vi "All Unsafe Config.vi"() -> (2 "All Unsafe Config":T1={"Inspections (All)"=[], "Disallowed ClassNames"=["Open Data Storage", "PathConstant", "Constructor", "Python Node", "Call MATLAB Function"], "Disallowed Functions"=[], "Disallowed SubVI Paths"=[], "Allowed Properties"=["VI Name"], "Allowed Invoke Nodes"=[]})   [LabVIEW 2020, in "SoL Inspector.lvlib"]
uses:
  SoL Inspector.lvlib
  Inspector Config.ctl
  Inspection.ctl
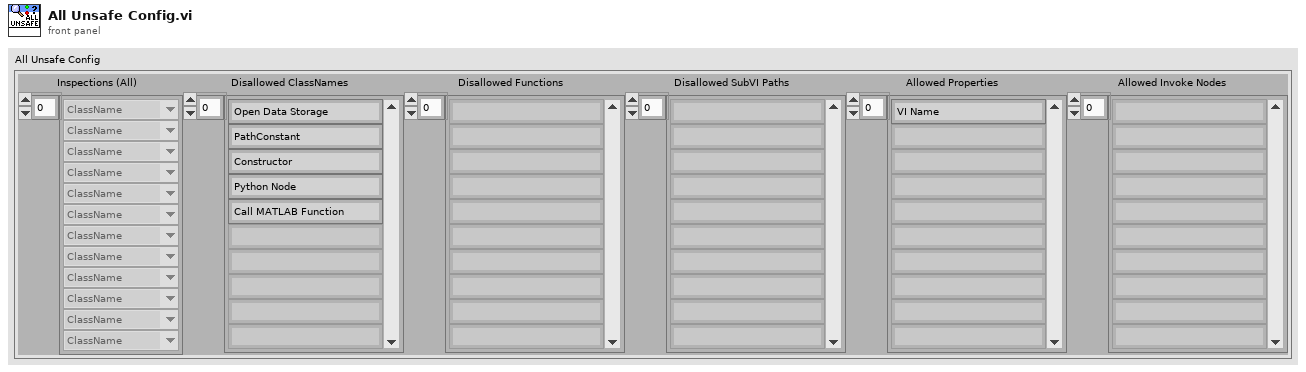
[diagram p1: front panel]
types:
  T1 = typedef "SoL Inspector.lvlib/Inspector Config.ctl" = cluster{"Inspections (All)":T2[], "Disallowed ClassNames":string[], "Disallowed Functions":string[], "Disallowed SubVI Paths":string[], "Allowed Properties":string[], "Allowed Invoke Nodes":string[]}
  T2 = typedef "SoL Inspector.lvlib/Inspection.ctl" = enum16{"ClassName", "Functions", "CallLibrary", "SubVIs", "FileIO", "Invoke Nodes", "Properties", "Growable Functions"}
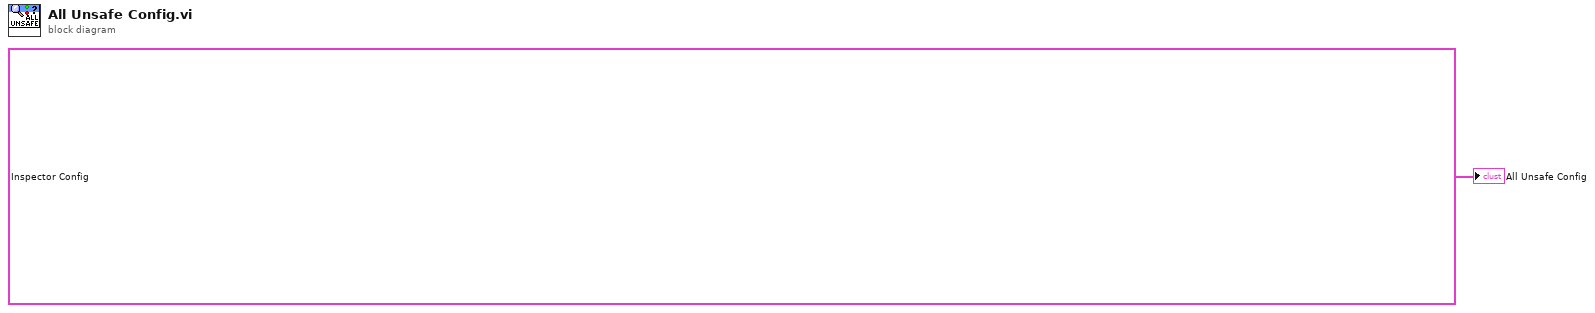
[diagram p0: block diagram]
diagram:
  "All Unsafe Config" <- T1 {"Inspections (All)"=[], "Disallowed ClassNames"=["Open Data Storage", "PathConstant", "Constructor", "Python Node", "Call MATLAB Function"], "Disallowed Functions"=["Open/Create/Replace File", "TCP Open Connection", "Close File", "Read from Binary File", "Write to Binary File", "Read from Text File", "Write to Text File", "TDMS Open", "New VI Object", "Open VI Object Reference", "New VI", "Call Chain", "Quit LabVIEW", "Stop", "Open Application Reference", "Open/Create/Replace Datalog", "Set Type and Creator", "Set File Size", "Set Permissions", "Delete", "Copy", "Move", "File/Directory Info", "Get Volume Info", "List Folder", "Create Folder", "Current VI's Path", "Temporary Directory", "Default Directory", "DataSocket Close", "DataSocket Open", "DataSocket Write", "DataSocket Read", "Create Network Stream Reader Endpoint", "Create Network Stream Writer Endpoint", "IP To String", "String To IP", "TCP Create Listener", "TCP Open Connection", "Load Private Key Into Memory", "Load Certificates Into Memory", "UDP Open", "VISA Read", "VISA Write", "IrDA Create Listener", "IrDA Open Connection", "IrDA Discover", "Bluetooth Discover", "Bluetooth Create Listener", "Bluetooth Open Connection", "Automation Open", "Open Python Session", "Open MATLAB Session", "Strip Path", "Build Path", "Array of Strings to Path", "String To Path"], "Disallowed SubVI Paths"=["C:\\Program Files (x86)\\National Instruments\\LabVIEW 2024\\vi.lib\\Utility\\file.llb\\", "C:\\Program Files (x86)\\National Instruments\\LabVIEW 2024\\vi.lib\\Utility\\config.llb\\", "C:\\Program Files (x86)\\National Instruments\\LabVIEW 2024\\vi.lib\\zip\\", "C:\\Program Files (x86)\\National Instruments\\LabVIEW 2024\\vi.lib\\Utility\\SystemLogging\\", "C:\\Program Files (x86)\\National Instruments\\LabVIEW 2024\\vi.lib\\Utility\\cursorutil.llb\\", "C:\\Program Files (x86)\\National Instruments\\LabVIEW 2024\\vi.lib\\Waveform\\WDTFileIO.llb\\", "C:\\Program Files (x86)\\National Instruments\\LabVIEW 2024\\vi.lib\\Platform\\storage\\utility\\", "C:\\Program Files (x86)\\National Instruments\\LabVIEW 2024\\vi.lib\\xml\\", "C:\\Program Files (x86)\\National Instruments\\LabVIEW 2024\\vi.lib\\Utility\\xml.llb\\", "C:\\Program Files (x86)\\National Instruments\\LabVIEW 2024\\vi.lib\\Utility\\sysdir.llb\\", "C:\\Program Files (x86)\\National Instruments\\LabVIEW 2024\\vi.lib\\Utility\\LVClass\\", "C:\\Program Files (x86)\\National Instruments\\LabVIEW 2024\\vi.lib\\picture\\bmp.llb\\", "C:\\Program Files (x86)\\National Instruments\\LabVIEW 2024\\vi.lib\\picture\\png.llb\\", "C:\\Program Files (x86)\\National Instruments\\LabVIEW 2024\\vi.lib\\picture\\jpeg.llb\\", "C:\\Program Files (x86)\\National Instruments\\LabVIEW 2024\\vi.lib\\Platform\\system.llb\\", "C:\\Program Files (x86)\\National Instruments\\LabVIEW 2024\\vi.lib\\sound2\\lvsound2.llb\\", "C:\\Program Files (x86)\\National Instruments\\LabVIEW 2024\\vi.lib\\picture\\3D Picture Control\\File Loading\\", "C:\\Program Files (x86)\\National Instruments\\LabVIEW 2024\\vi.lib\\Utility\\NIReport.llb\\", "C:\\Program Files (x86)\\National Instruments\\LabVIEW 2024\\vi.lib\\AppBuilder\\", "C:\\Program Files (x86)\\National Instruments\\LabVIEW 2024\\vi.lib\\Utility\\traverseref.llb\\", "C:\\Program Files (x86)\\National Instruments\\LabVIEW 2024\\vi.lib\\MemoryControl\\", "C:\\Program Files (x86)\\National Instruments\\LabVIEW 2024\\vi.lib\\Palette API\\", "C:\\Program Files (x86)\\National Instruments\\LabVIEW 2024\\vi.lib\\Utility\\Get Command Line Arguments.vi", "C:\\Program Files\\NI\\LVAddons\\viawin\\1\\vi.lib\\addons\\analyzer\\analyzerapi.llb\\", "C:\\Program Files\\NI\\LVAddons\\utf32\\1\\vi.lib\\utf\\", "C:\\Program Files (x86)\\National Instruments\\LabVIEW 2024\\vi.lib\\Utility\\LVLibp\\", "C:\\Program Files (x86)\\National Instruments\\LabVIEW 2024\\vi.lib\\Utility\\libraryn.llb\\", "C:\\Program Files (x86)\\National Instruments\\LabVIEW 2024\\vi.lib\\security\\Message Digest\\", "C:\\Program Files (x86)\\National Instruments\\LabVIEW 2024\\vi.lib\\Utility\\file.llb\\", "C:\\Program Files (x86)\\National Instruments\\LabVIEW 2024\\vi.lib\\Platform\\dataskt.llb\\", "C:\\Program Files (x86)\\National Instruments\\LabVIEW 2024\\vi.lib\\Utility\\Resolve Machine Alias.vi", "C:\\Program Files (x86)\\National Instruments\\LabVIEW 2024\\vi.lib\\Utility\\tcp.llb\\", "C:\\Program Files (x86)\\National Instruments\\LabVIEW 2024\\vi.lib\\Instr\\_visa.llb\\", "C:\\Program Files (x86)\\National Instruments\\LabVIEW 2024\\vi.lib\\Platform\\Bluetooth.llb\\", "C:\\Program Files (x86)\\National Instruments\\LabVIEW 2024\\vi.lib\\smtpClient\\", "C:\\Program Files (x86)\\National Instruments\\LabVIEW 2024\\vi.lib\\httpClient\\", "C:\\Program Files (x86)\\National Instruments\\LabVIEW 2024\\vi.lib\\FTP\\", "C:\\Program Files (x86)\\National Instruments\\LabVIEW 2024\\vi.lib\\WebDAVClient\\", "C:\\Program Files (x86)\\National Instruments\\LabVIEW 2024\\vi.lib\\net\\", "C:\\Program Files (x86)\\National Instruments\\LabVIEW 2024\\vi.lib\\SourceControl\\", "C:\\Program Files (x86)\\National Instruments\\LabVIEW 2024\\vi.lib\\wsapi\\", "C:\\Program Files (x86)\\National Instruments\\LabVIEW 2024\\vi.lib\\Platform\\dotnet.llb\\", "C:\\Program Files (x86)\\National Instruments\\LabVIEW 2024\\vi.lib\\Utility\\inputDevices.llb\\", "C:\\Program Files (x86)\\National Instruments\\LabVIEW 2024\\vi.lib\\registry\\", "C:\\Program Files (x86)\\National Instruments\\LabVIEW 2024\\vi.lib\\Python\\", "C:\\Program Files\\NI\\LVAddons\\dct\\1\\vi.lib\\addons\\database\\", "C:\\Program Files\\NI\\LVAddons\\dfc\\1\\vi.lib\\DataFinder\\", "C:\\Program Files (x86)\\National Instruments\\LabVIEW 2024\\vi.lib\\MakerHub\\", "C:\\Program Files\\NI\\LVAddons\\nisyscfg\\1\\vi.lib\\nisyscfg\\"], "Allowed Properties"=["VI Name"], "Allowed Invoke Nodes"=[]} ("Inspector Config")
